vi "Add Report Information.vi"(8 "error in (no error)":errorcluster, 10 "Report Information.lvclass":refnum<class "Report Information.lvclass">, 11 "OnTheFlyReport in":refnum<class "OnTheFlyReport.lvclass">) -> (0 "error out":errorcluster, 3 "OnTheFlyReport out":refnum<class "OnTheFlyReport.lvclass">)   [LabVIEW 2015, in "OnTheFlyReport.lvclass"]
doc: "This VI takes an entire Result Information object and saves it to the permanent report."
uses:
  OnTheFlyReport.lvclass
  Report Information/Report Information.lvclass
  OnTheFlyReport.lvclass/OnTheFlyReport.ctl
  Report Formatters/Base Class/Formatter.lvclass
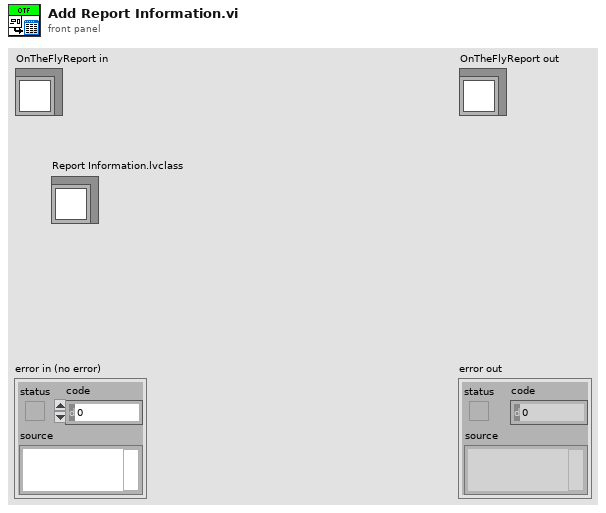
[diagram p1: front panel]
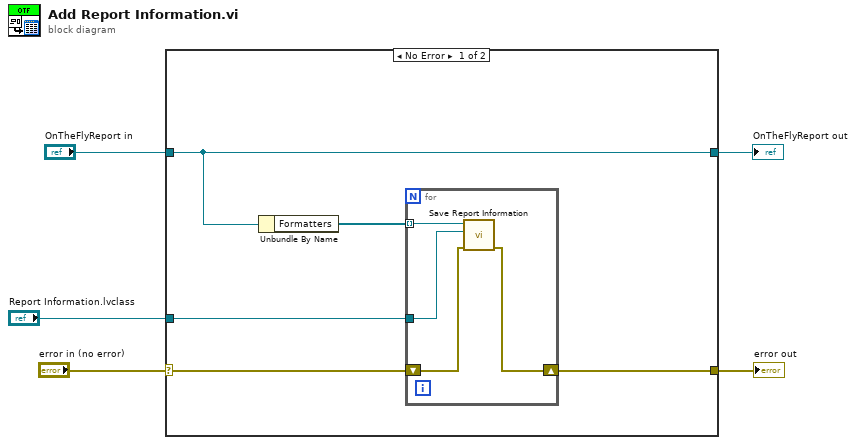
[diagram p0: block diagram]
diagram:
  n1 = case shown="No Error" "error in (no error)" {
    selector: "error in (no error)" -> [w8 w16]
    tunnel: [w7 w16] -> w5
    tunnel: [w6 w15] -> w4
    tunnel: "OnTheFlyReport in" -> [w6 w15]
    tunnel: "Report Information.lvclass" -> [w9 _]
    frame No Error {
      n2 = Unbundle By Name(w6) -> ("Formatters"=w10:refnum<class "Formatter.lvclass">[])
      n3 = for {
        tunnel: w10 -> [w14] mode=indexing
        tunnel: w9 -> [w11]
        shift-right: [w12] -> w7
        shift-left: w8 -> [w13]
        n4 = call-dynamic "Save Report Information.vi"("error in (no error)"=w13, "Report Information.lvclass"=w11, "Formatter in"=w14) -> ("error out"=w12:errorcluster)  [unwired: 7 in, 1 out]
      }
    }
    frame Error {
    }
  }
  "error out" <- w5
  "OnTheFlyReport out" <- w4
